vi "ProcessWfm.vi"(8 "low cutoff freq: fl":dbl=0.001 format="%#_13g", 9 "high cutoff freq: fh":dbl=1000.0 format="%#_13g", 10 "Delay (bins)":dbl, 11 "Waveform":waveform(dbl)) -> (3 "Delayed Filtered waveform":waveform(dbl))   [LabVIEW 2011]
uses:
  <vilib>/Analysis/NI_AALBase.lvlib
  <vilib>/Analysis/3filter.llb/Butterworth Filter (DBL).vi
  <vilib>/Analysis/3filter.llb/Filter Passband Type.ctl
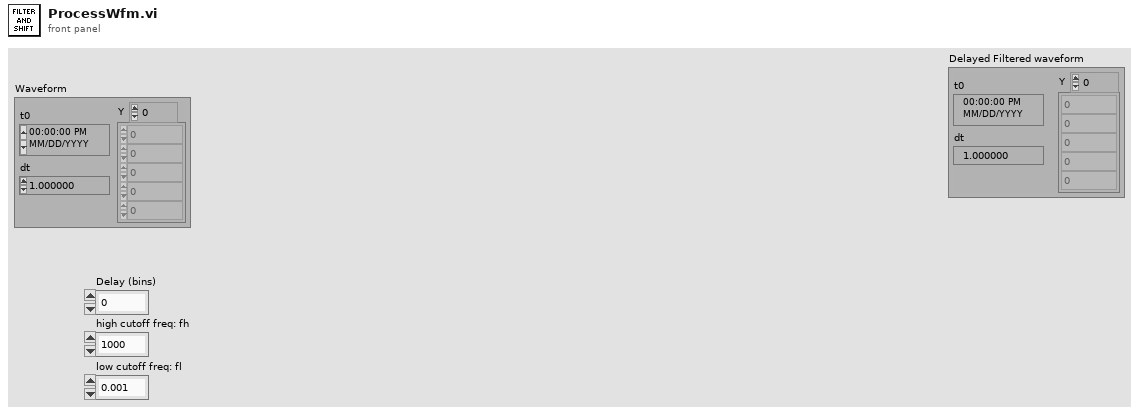
[diagram p1: front panel]
types:
  T1 = typedef "NI_AALBase.lvlib/Filter Passband Type.ctl" = enum32{"Lowpass", "Highpass", "Bandpass", "Bandstop"}
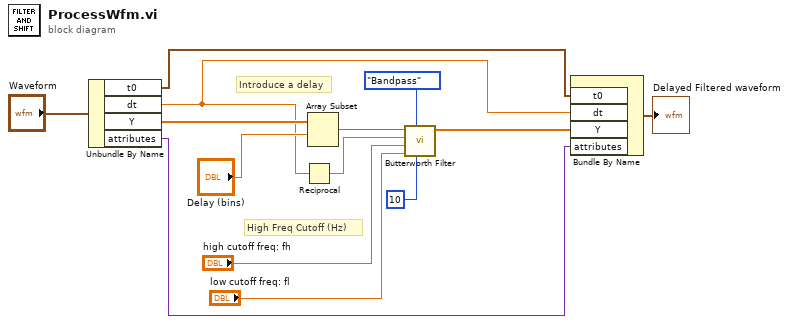
[diagram p0: block diagram]
diagram:
  # "High Freq Cutoff (Hz)"
  # "Introduce a delay"
  n1 = Unbundle By Name("Waveform") -> ("t0"=w6:timestamp, "dt"=w2:dbl, "Y"=w13:dbl[], "attributes"=w5:variant)
  n2 = Reciprocal(x=w2) -> (1/x=w1:dbl)
  n3 = Array Subset(array=w13, index="Delay (bins)") -> (w11:dbl[])  [unwired: 1 in]
  n4 = call-poly <vilib>:"Butterworth Filter.vi"("order"=10, "filter type"=Filter_Passband_Type."Bandpass", "low cutoff freq: fl"="low cutoff freq: fl", "high cutoff freq: fh"="high cutoff freq: fh", "sampling freq: fs"=w1, "X"=w11) -> ("Filtered X"=w7:dbl[])  [unwired: 2 in, 1 out]
  n5 = Bundle By Name("t0"=w6, "dt"=w2, "Y"=w7, "attributes"=w5) -> (→"Delayed Filtered waveform":waveform(dbl))  [unwired: 1 in]
